vi "EXCOM_25.vi"(0 "VISA resource name":refnum<visa-resource-name>) -> (5 "OK Done":bool, 6 "HA":dbl format="%<%H:%M:%S%0u>t", 7 "Q String":string, 8 "RA":dbl format="%<%H:%M:%S%0u>t", 9 "Rotateur":dbl format="%.2f", 10 "DEC":dbl format="%<%H:%M:%S%0u>t", 11 "Dome":dbl format="%.2f", 12 "Epoque":dbl format="%.2f", 13 "Focus":dbl format="%.2f", 14 "VISA resource name dup":refnum<visa-resource-name>, 15 "Masse d'air":dbl format="%.2f", 16 "Temps Sidéral":dbl format="%<%H:%M:%S%0u>t", 17 "Temps Universel":dbl format="%<%H:%M:%S%0u>t", 18 "Année":dbl format="%.2f", 19 "Error OUT":errorcluster)   [LabVIEW 2011]
panel:
  out "ExecTime":u32
  in  "Error IN":errorcluster
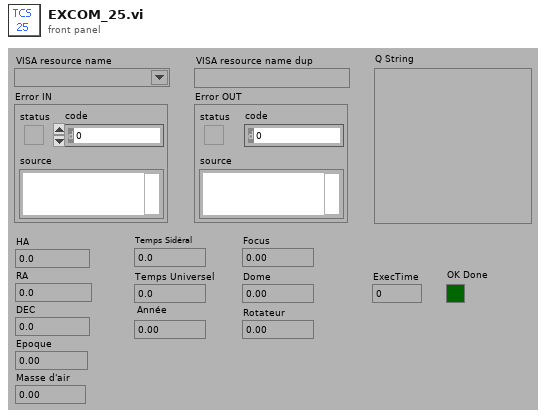
[diagram p1: front panel]
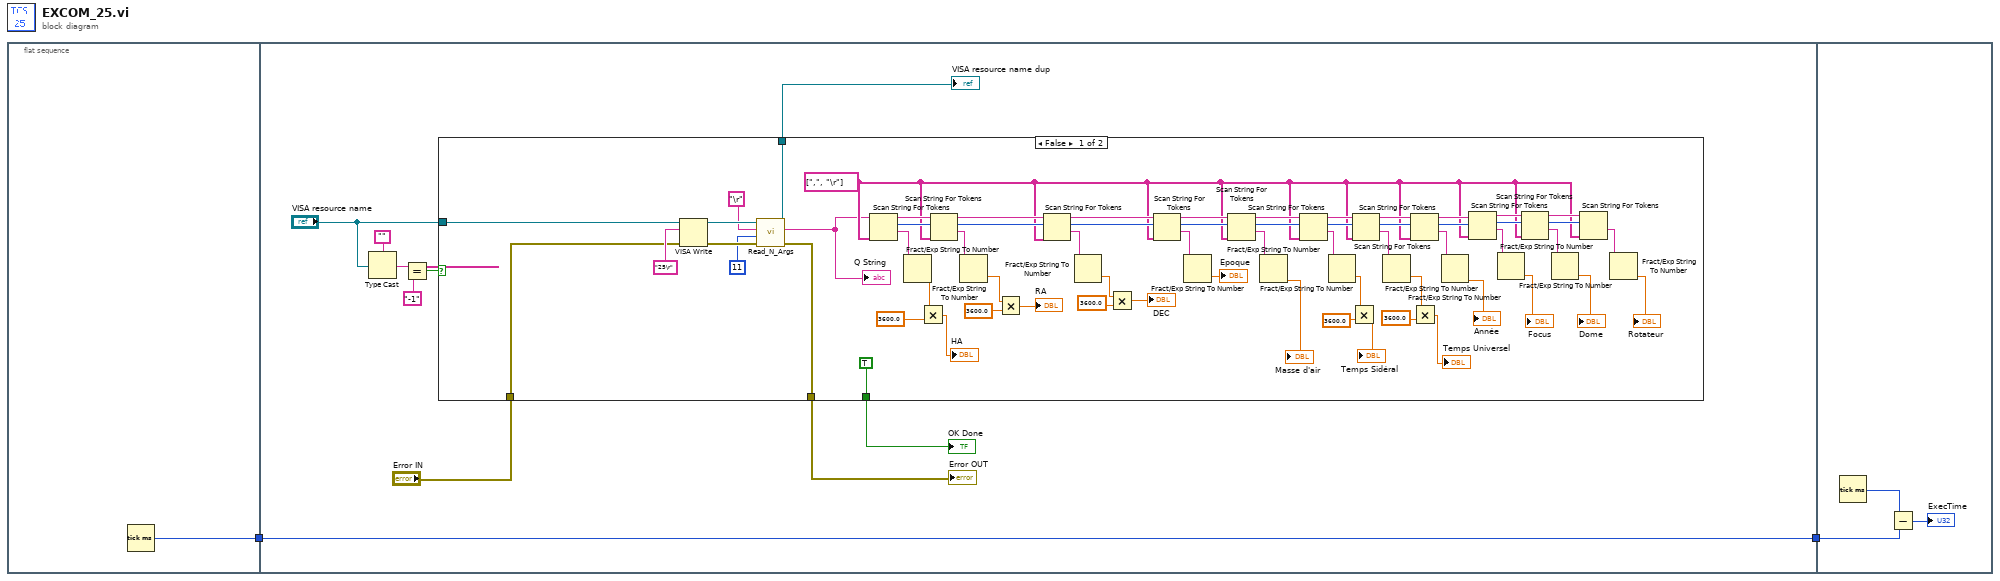
[diagram p0: block diagram]
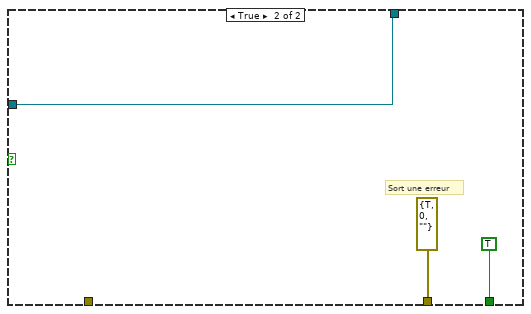
[diagram p2: hidden frame]
diagram:
  n1 = flat-sequence {
    tunnel: [w3] -> w2
    tunnel: w2 -> [w5]
    tunnel: [w5] -> w1
    tunnel: w1 -> [w83]
    frame #0 {
      n2 = Tick Count (ms)() -> (millisecond timer value=w3:u32)
    }
    frame #1 {
      n3 = Type Cast(type="", x="VISA resource name") -> (*(type *) &x=w12:string)
      n4 = Equal?(x=w12, y="-1") -> (x = y?=w10:bool)
      n5 = case shown="False" w10 {
        tunnel: "VISA resource name" -> [w15 w78]
        tunnel: [TRUE ("OK Done") TRUE ("OK Done")] -> w8
        tunnel: [w22 errorcluster {"status"=TRUE, "code"=0, "source"=""} ("error out")] -> w7
        tunnel: [w16 w78] -> w6
        tunnel: "Error IN" -> [w14 _]
        frame False {
          w26 = string[] [",", "\r"] ("delimiters (\\s,\\t,\\r,\\n)")
          n6 = VISA Write(VISA resource name=w15, write buffer="25\r" ("String to Send"), error in (no error)=w14) -> (VISA resource name out=w20:refnum<visa-resource-name>, error out=w21:errorcluster)  [unwired: 1 out]
          n7 = call "Read_N_Args.vi"("Error IN"=w21, "Nb_Args"=11, "Arg_Char"="\r", "VRN IN"=w20) -> ("Error OUT"=w22:errorcluster, "Answer"=w23:string, "VRN OUT"=w16:refnum<visa-resource-name>)  [unwired: 4 in, 1 out]
          "Q String" <- w23
          n8 = Scan String For Tokens(6:w26, 9:w23) -> (1:w69:string, 2:w70:i32, 3:w71:string)  [unwired: 4 in, 1 out]
          n9 = Fract/Exp String To Number(string=w69) -> (number=w68:dbl)  [unwired: 3 in, 1 out]
          n10 = Multiply(x=w68, y=3600.0) -> (x*y=→"HA":dbl)
          n11 = Scan String For Tokens(6:w26, 8:w70, 9:w71) -> (1:w27:string, 2:w73:i32, 3:w72:string)  [unwired: 3 in, 1 out]
          n12 = Fract/Exp String To Number(string=w27) -> (number=w60:dbl)  [unwired: 3 in, 1 out]
          n13 = Multiply(x=w60, y=3600.0) -> (x*y=→"RA":dbl)
          n14 = Scan String For Tokens(6:w26, 8:w73, 9:w72) -> (1:w63:string, 2:w75:i32, 3:w74:string)  [unwired: 3 in, 1 out]
          n15 = Fract/Exp String To Number(string=w63) -> (number=w58:dbl)  [unwired: 3 in, 1 out]
          n16 = Multiply(x=w58, y=3600.0) -> (x*y=→"DEC":dbl)
          n17 = Scan String For Tokens(6:w26, 8:w75, 9:w74) -> (1:w62:string, 2:w77:i32, 3:w76:string)  [unwired: 3 in, 1 out]
          n18 = Fract/Exp String To Number(string=w62) -> (number=→"Epoque":dbl)  [unwired: 3 in, 1 out]
          n19 = Scan String For Tokens(6:w26, 8:w77, 9:w76) -> (1:w61:string, 2:w29:i32, 3:w48:string)  [unwired: 3 in, 1 out]
          n20 = Fract/Exp String To Number(string=w61) -> (number=→"Masse d'air":dbl)  [unwired: 3 in, 1 out]
          n21 = Scan String For Tokens(6:w26, 8:w29, 9:w48) -> (1:w53:string, 2:w51:i32, 3:w52:string)  [unwired: 3 in, 1 out]
          n22 = Fract/Exp String To Number(string=w53) -> (number=w56:dbl)  [unwired: 3 in, 1 out]
          n23 = Multiply(x=w56, y=3600.0) -> (x*y=→"Temps Sidéral":dbl)
          n24 = Scan String For Tokens(6:w26, 8:w51, 9:w52) -> (1:w54:string, 2:w49:i32, 3:w50:string)  [unwired: 3 in, 1 out]
          n25 = Fract/Exp String To Number(string=w54) -> (number=w57:dbl)  [unwired: 3 in, 1 out]
          n26 = Scan String For Tokens(6:w26, 8:w49, 9:w50) -> (1:w55:string, 2:w28:i32, 3:w38:string)  [unwired: 3 in, 1 out]
          n27 = Multiply(x=w57, y=3600.0) -> (x*y=→"Temps Universel":dbl)
          n28 = Fract/Exp String To Number(string=w55) -> (number=→"Année":dbl)  [unwired: 3 in, 1 out]
          n29 = Scan String For Tokens(6:w26, 8:w28, 9:w38) -> (1:w41:string, 2:w43:i32, 3:w42:string)  [unwired: 3 in, 1 out]
          n30 = Fract/Exp String To Number(string=w41) -> (number=→"Focus":dbl)  [unwired: 3 in, 1 out]
          n31 = Scan String For Tokens(6:w26, 8:w43, 9:w42) -> (1:w40:string, 2:w45:i32, 3:w44:string)  [unwired: 3 in, 1 out]
          n32 = Fract/Exp String To Number(string=w40) -> (number=→"Dome":dbl)  [unwired: 3 in, 1 out]
          n33 = Scan String For Tokens(6:w26, 8:w45, 9:w44) -> (1:w39:string)  [unwired: 3 in, 3 out]
          n34 = Fract/Exp String To Number(string=w39) -> (number=→"Rotateur":dbl)  [unwired: 3 in, 1 out]
        }
        frame True {
          # "Sort une erreur"
        }
      }
      "VISA resource name dup" <- w6
      "OK Done" <- w8
      "Error OUT" <- w7
    }
    frame #2 {
      n35 = Tick Count (ms)() -> (millisecond timer value=w82:u32)
      n36 = Subtract(x=w82, y=w83) -> (x-y=→"ExecTime":u32)
    }
  }
